vi "Z_CONT.vi"(8 "error in (no error)":errorcluster, 9 "element":T1 {"Avoid zero threshold (V)" format="%#_13g"}, 10 "ScanQ in":refnum<queue>, 11 "Queue in":refnum<queue>) -> (0 "error out":errorcluster, 2 "Z-Controller on/off status":bool, 3 "Queue out":refnum<queue>)   [LabVIEW 2025]
uses:
  <userlib>/Nanonis Prog Interface V5e/Nanonis Prog Interface.lvlib
  Labview-File/STM-Auto-Project Testing/STM-Auto-Project (Trial 2)/QMH CTLS/Scan_Params (QMH).ctl
  Temp Cntrl.ctl
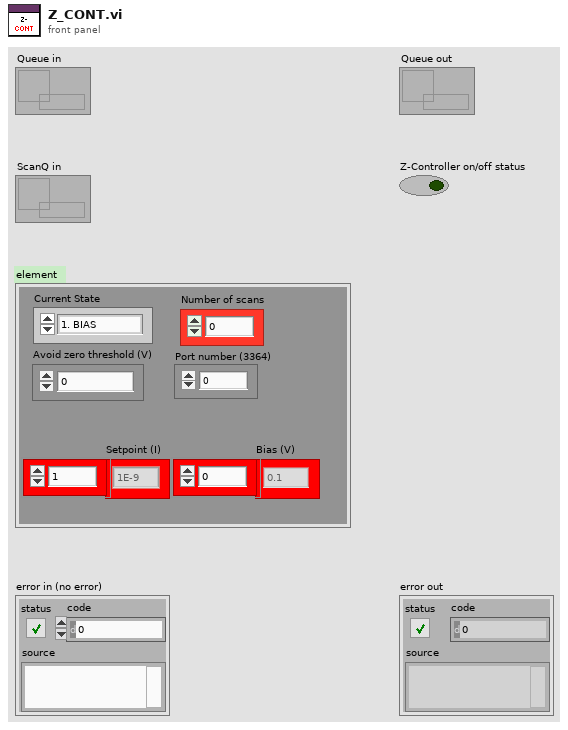
[diagram p1: front panel]
types:
  T1 = typedef "Scan_Params (QMH).ctl" = cluster{"Setpoint (I)":dbl[], "Bias (V)":dbl[], "Number of scans":u8, "Port number (3364)":u32, "Avoid zero threshold (V)":dbl, "Current State":enum16{"1. BIAS", "2. INIT_SCAN", "3. SCAN_IDLE", "4. INTER_SCAN", "5. NEW_COORDS_&_FRAME", "6. FINAL_SCAN", "7. STOP"}}
  T2 = enum16{"1. BIAS", "2. INIT_SCAN", "3. SCAN_IDLE", "4. INTER_SCAN", "5. NEW_COORDS_&_FRAME", "6. FINAL_SCAN", "7. POLL_BIAS", "8. Z-CONT.", "9. STOP"}
  T3 = enum16{"1. INIT TEMP", "2. TC ON", "3. POLL_TEMPS", "4. TEMP_STAB", "5. TC IDLE", "6. APPLY NEXT TEMP", "7. TC OFF (Reset)"}
  T4 = typedef "Temp Cntrl.ctl" = cluster{"Range (0:Off)":u16, "Manual Output (0.00 %)":dbl, "Rate (D) (0.0 %)":dbl, "Reset (I) (20.0)":dbl, "Gain (P) (50.0)":dbl, "Power Up Enable (F: Disable)":bool, "Max User Current (2.000)":dbl, "Heater Resistance (1:25 Ohms)":u16, "Max Current (0:User Specified)":u16, "Heater Out Display (1:Current)":u16, "Mode (0:Off)":u16, "Input (0:None)":u16, "Target Temp (K)":dbl, "Serial Configuration":cluster{"Baud Rate":u32, "Parity":u16, "Data Bits":u16, "Stop Bits":u16, "Flow Control":u16}, "VISA resource name":refnum<visa-resource-name>, "Configure Control Parameters (0: Configure)":u16, "Enable Setpoint (F:Disable)":bool, "Input (0:A)":u16, "Data Source (0:Kelvin)":u16, "Output's Control Loop (1:1)":u16, "STND DEV Threshold ":dbl, "Mean Tolerance ":dbl, "Current State":enum16{"1. INIT TEMP", "2. TC ON", "3. POLL_TEMPS", "4. TEMP_STAB", "5. TC IDLE", "6. APPLY NEXT TEMP", "7. TC OFF (Reset)"}}
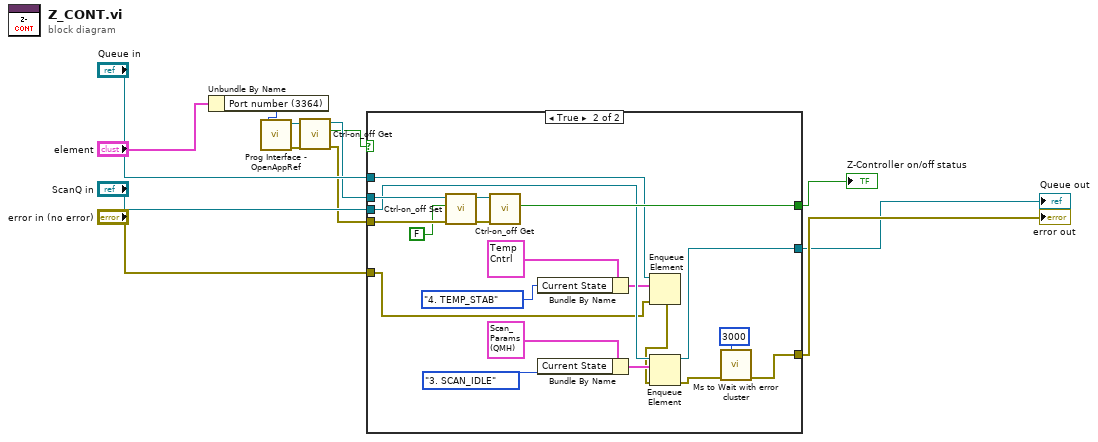
[diagram p0: block diagram]
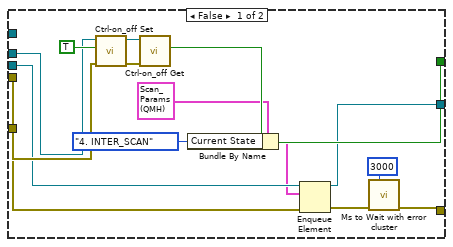
[diagram p2: hidden frame]
diagram:
  n1 = Unbundle By Name("element") -> ("Port number (3364)"=w13:u32)
  n2 = call <userlib>:"Prog Interface - OpenAppRef.vi"("Port number (3364)"=w13) -> ("Error out"=w10:errorcluster, "Application reference"=w11:refnum<vi>)  [unwired: 5 in]
  n3 = call <userlib>:"Ctrl-on_off Get.vi"("error in (no error)"=w10, "Application ref in"=w11) -> ("error out"=w3:errorcluster, "Z-Controller on/off status"=w1:bool, "Application ref out"=w2:refnum<vi>)  [unwired: 7 in]
  n4 = case shown="True" w1 {
    tunnel: w2 -> [w25 w48]
    tunnel: w3 -> [w24 w47]
    tunnel: [w23 w43] -> w4
    tunnel: "ScanQ in" -> [w22 w42]
    tunnel: [w19 w39] -> w6
    tunnel: [w15 w29] -> w7
    tunnel: "error in (no error)" -> [w18 w34]
    tunnel: "Queue in" -> [_ w38]
    frame False {
      n5 = call <userlib>:"Ctrl-on_off Set.vi"("error in (no error)"=w24, "Z Controller ON/OFF"=TRUE, "Application ref in"=w25) -> ("error out"=w27:errorcluster, "Application ref out"=w26:refnum<vi>)  [unwired: 7 in]
      n6 = call <userlib>:"Ctrl-on_off Get.vi"("error in (no error)"=w27, "Application ref in"=w26) -> ("Z-Controller on/off status"=w23:bool)  [unwired: 7 in, 2 out]
      n7 = Bundle By Name(cluster=T1 {"Setpoint (I)"=[], "Bias (V)"=[], "Number of scans"=1, "Port number (3364)"=3364, "Avoid zero threshold (V)"=0.004999999888241291, "Current State"=enum."1. BIAS"} ("element"), "Current State"=T2."4. INTER_SCAN") -> (w20:T1)
      n8 = Enqueue Element(queue=w22, element=w20, error in (no error)=w18) -> (queue out=w19:refnum<queue>, error out=w16:errorcluster)  [unwired: 1 in, 1 out]
      n9 = call <userlib>:"Ms to Wait with error cluster.vi"("error in (no error)"=w16, "milliseconds to wait"=u32 3000) -> ("error out"=w15:errorcluster)  [unwired: 4 in, 1 out]
    }
    frame True {
      n10 = call <userlib>:"Ctrl-on_off Set.vi"("error in (no error)"=w47, "Z Controller ON/OFF"=FALSE, "Application ref in"=w48) -> ("error out"=w45:errorcluster, "Application ref out"=w44:refnum<vi>)  [unwired: 7 in]
      n11 = call <userlib>:"Ctrl-on_off Get.vi"("error in (no error)"=w45, "Application ref in"=w44) -> ("Z-Controller on/off status"=w43:bool)  [unwired: 7 in, 2 out]
      n12 = Bundle By Name(cluster=T4 {"Range (0:Off)"=0, "Manual Output (0.00 %)"=0.0, "Rate (D) (0.0 %)"=0.0, "Reset (I) (20.0)"=20.0, "Gain (P) (50.0)"=50.0, "Power Up Enable (F: Disable)"=FALSE, "Max User Current (2.000)"=2.0, "Heater Resistance (1:25 Ohms)"=1, "Max Current (0:User Specified)"=0, "Heater Out Display (1:Current)"=1, "Mode (0:Off)"=1, "Input (0:None)"=4, "Target Temp (K)"=5.0, "Serial Configuration"={"Baud Rate"=57600, "Parity"=1, "Data Bits"=7, "Stop Bits"=10, "Flow Control"=0}, "VISA resource name"="", "Configure Control Parameters (0: Configure)"=0, "Enable Setpoint (F:Disable)"=FALSE, "Input (0:A)"=3, "Data Source (0:Kelvin)"=0, "Output's Control Loop (1:1)"=2, "STND DEV Threshold "=0.1, "Mean Tolerance "=0.02, "Current State"=enum."1. INIT TEMP"} ("element"), "Current State"=T3."4. TEMP_STAB") -> (w37:T4)
      n13 = Bundle By Name(cluster=T1 {"Setpoint (I)"=[], "Bias (V)"=[], "Number of scans"=1, "Port number (3364)"=3364, "Avoid zero threshold (V)"=0.004999999888241291, "Current State"=enum."1. BIAS"} ("element"), "Current State"=T2."3. SCAN_IDLE") -> (w40:T1)
      n14 = Enqueue Element(queue=w38, element=w37, error in (no error)=w34) -> (error out=w33:errorcluster)  [unwired: 1 in, 2 out]
      n15 = Enqueue Element(queue=w42, element=w40, error in (no error)=w33) -> (queue out=w39:refnum<queue>, error out=w30:errorcluster)  [unwired: 1 in, 1 out]
      n16 = call <userlib>:"Ms to Wait with error cluster.vi"("error in (no error)"=w30, "milliseconds to wait"=u32 3000) -> ("error out"=w29:errorcluster)  [unwired: 4 in, 1 out]
    }
  }
  "error out" <- w7
  "Queue out" <- w6
  "Z-Controller on/off status" <- w4
